vi "ByRef1_Create.vi"(8 "error in (no error)":errorcluster, 11 "reference in":refnum<class "ByRef1.lvclass">) -> (0 "error out":errorcluster, 3 "reference out":refnum<class "ByRef1.lvclass">)   [LabVIEW 2020, in "ByRef1.lvclass"]
uses:
  ByRef1.lvclass
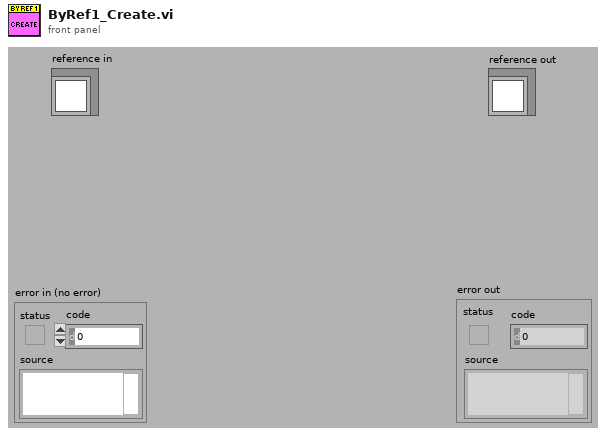
[diagram p1: front panel]
types:
  T1 = typedef "ByRef1.lvclass/ObjectAttributes.ctl" = cluster{"Triggers":i32}
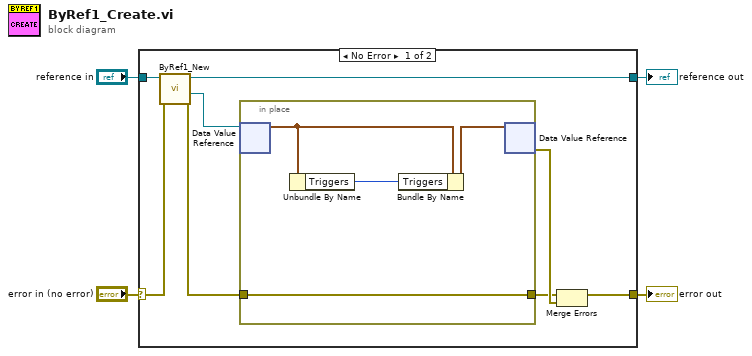
[diagram p0: block diagram]
diagram:
  n1 = case shown="No Error" "error in (no error)" {
    selector: "error in (no error)" -> [w11 w18]
    tunnel: [w5 w18] -> w3
    tunnel: "reference in" -> [w12 w17]
    tunnel: [w10 w17] -> w1
    frame No Error {
      n2 = call "ByRef1_New.vi"("error in (no error)"=w11, "reference in"=w12) -> ("error out"=w7:errorcluster, "DVRRefOut"=w8:refnum<data-value>, "reference out"=w10:refnum<class "ByRef1.lvclass">)  [unwired: 6 in, 1 out]
      n3 = in-place {
        in-place-border: w7 -> [w13]
        in-place-border: [w13] -> w6
        n4 = in-place-dvr #1(w8) -> (w15:T1)  [unwired: 1 out]
        n5 = Unbundle By Name(w15) -> ("Triggers"=w14:i32)
        n6 = Bundle By Name(cluster=w15, "Triggers"=w14) -> (w16:T1)
        n7 = in-place-dvr #1(w16) -> (w9:errorcluster)  [unwired: 1 out]
      }
      n8 = Merge Errors(w6, w9) -> (w5:errorcluster)
    }
    frame Error {
      # "VI-TechBaseTemplate_Simple_4x4x4"
    }
  }
  "error out" <- w3
  "reference out" <- w1
